vi "SC TCP Send Command and Wait for Response.vi"(8 "error in (no error)":errorcluster, 9 "timeout (10000 ms)":i32=10000, 10 "Command":string, 11 "TCP Network Connection in":refnum<k5>) -> (0 "error out":errorcluster, 1 "Timed Out":bool, 2 "Response":string, 3 "TCP Network Connection out":refnum<k5>)   [LabVIEW 2018]
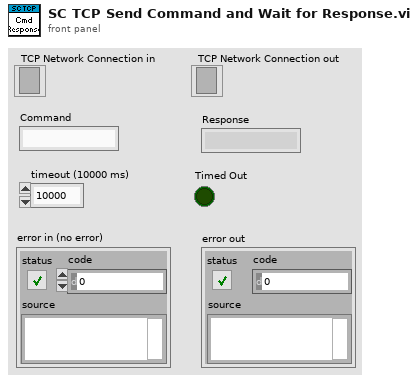
[diagram p1: front panel]
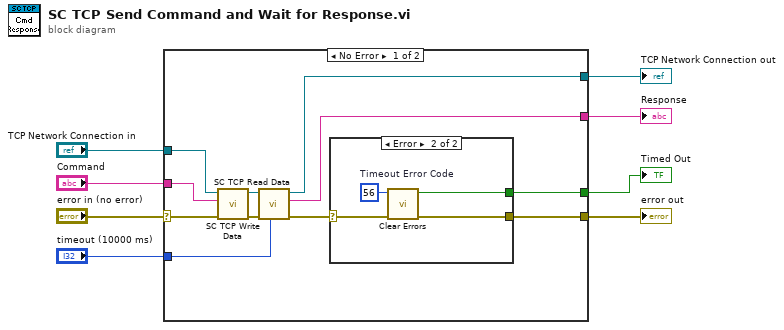
[diagram p0: block diagram]
diagram:
  n1 = case shown="No Error" "error in (no error)" {
    selector: "error in (no error)" -> [w11 w26]
    tunnel: [w19 _] -> w8
    tunnel: "timeout (10000 ms)" -> [w18 _]
    tunnel: "TCP Network Connection in" -> [w17 w25]
    tunnel: "Command" -> [w16 _]
    tunnel: [w15 _] -> w4
    tunnel: [w10 w26] -> w2
    tunnel: [w9 w25] -> w1
    frame No Error {
      n2 = call "SC TCP Write Data.vi"("error in"=w11, "Data"=w16, "TCP Network Connection in"=w17) -> ("error out"=w14:errorcluster, "TCP Network Connection out"=w13:refnum<k5>)  [unwired: 7 in]
      n3 = call "SC TCP Read Data.vi"("timeout ms (25000)"=w18, "error in"=w14, "TCP  Connection in"=w13) -> ("error out"=w12:errorcluster, "data"=w19:string, "TCP  Connection out"=w9:refnum<k5>)  [unwired: 6 in]
      n4 = case shown="Error" w12 {
        selector: w12 -> [w20 w22]
        tunnel: [w20 w23] -> w10
        tunnel: [_ w21] -> w15
        frame No Error {
        }
        frame Error {
          w24 = 56  # Timeout Error Code
          n5 = call <vilib>:"Clear Errors.vi"("error in (no error)"=w22, "specific error code to clear (0: all)"=w24) -> ("error out"=w23:errorcluster, "specific error cleared?"=w21:bool)  [unwired: 4 in]
        }
      }
    }
    frame Error {
    }
  }
  "Response" <- w8
  "error out" <- w2
  "Timed Out" <- w4
  "TCP Network Connection out" <- w1
